vi "visa test.vi"() -> ()   [LabVIEW 2022 SP3]
uses:
  <vilib>/Instr/_visa.llb/VISA Find Search Mode.ctl
  <vilib>/Instr/_visa.llb/VISA Configure Serial Port (Instr).vi
panel:
  in  "VISA resource name":refnum<visa-resource-name>
  in  "String":string
  out "error out":errorcluster
  out "Cfg":errorcluster
  in  "Index":i32
  out "find list":string[](array[string])
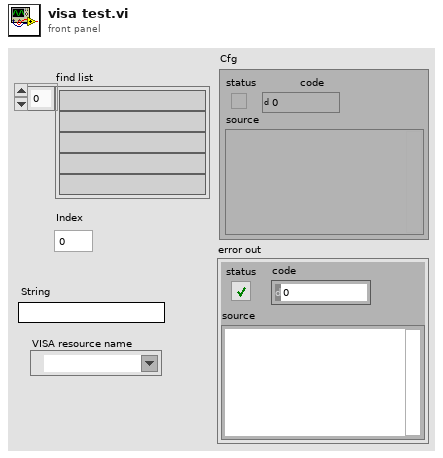
[diagram p1: front panel]
types:
  T1 = typedef "VISA Find Search Mode.ctl" = u32
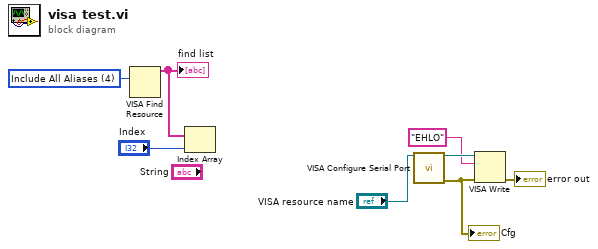
[diagram p0: block diagram]
diagram:
  w8 = T1 4 items=["Canonical Names Only"=0, "Aliases Only"=2, "Include Matching Aliases"=3, "Include All Aliases"=4] ("Search Mode")
  n1 = VISA Find Resource(10:w8) -> (3:w7:string[])  [unwired: 2 in, 2 out]
  "find list" <- w7
  n2 = Index Array(array=w7, index="Index") -> ()  [unwired: 1 out]
  n3 = call-poly "VISA Configure Serial Port"("VISA resource name"="VISA resource name") -> ("VISA resource name out"=w5:refnum<visa-resource-name>, "error out"=w4:errorcluster)  [unwired: 13 in]
  "Cfg" <- w4
  n4 = VISA Write(VISA resource name=w5, write buffer="EHLO", error in (no error)=w4) -> (error out=→"error out":errorcluster)  [unwired: 2 out]
